vi "Create FIFO Buffers.vi"(8 "error in (no error)":errorcluster) -> (0 "error out":errorcluster, 3 "FIFO Buffers":refnum<k33>[](array[refnum]))   [LabVIEW 2014]
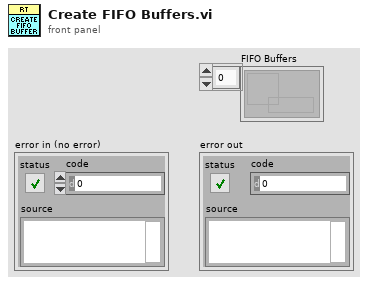
[diagram p1: front panel]
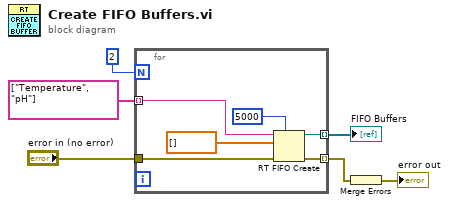
[diagram p0: block diagram]
diagram:
  n1 = for {
    N: 2 -> [_]
    tunnel: string[] ["Temperature", "pH"] -> [w11] mode=indexing
    tunnel: "error in (no error)" -> [w9]
    tunnel: [w8] -> w4 mode=indexing
    tunnel: [w7] -> w6 mode=indexing
    n2 = RT FIFO Create(0:w11, 1:dbl[] [], 3:w9, 4:u32 5000 ("size (10)")) -> (8:w7:refnum<k33>, 11:w8:errorcluster)  [unwired: 4 in, 1 out]
  }
  "FIFO Buffers" <- w6
  n3 = Merge Errors(w4) -> (→"error out":errorcluster)
